vi "CONF digital do task.vi"(6 "Route array":i32[](array[numeric])=[1, 2, 3, 4, 5, 6, 7, 8], 8 "error in (no error)":errorcluster, 9 "Reorder config (F)":bool=TRUE, 10 "AI HW conf array in":T1[](array[typedef]), 11 "Digital ref in":T2) -> (0 "error out":errorcluster, 2 "AI HW conf array out":T1[](array[typedef]), 3 "Digital ref out":T2)   [LabVIEW 2013]
uses:
  Kontrolki/KartaDAQ/CONF Digital Refnum.ctl
  Kontrolki/KartaDAQ/CONF AI HW config.ctl
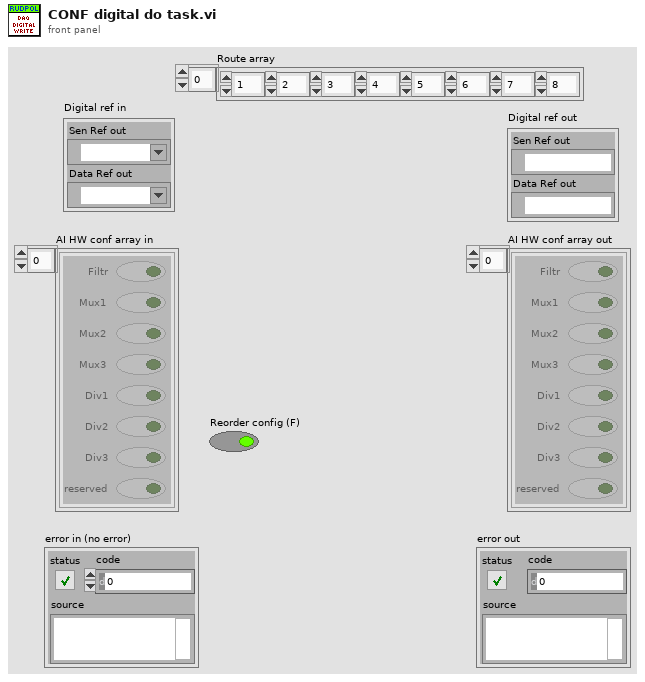
[diagram p1: front panel]
types:
  T1 = typedef "CONF AI HW config.ctl" = cluster{"Filtr":bool, "Mux1":bool, "Mux2":bool, "Mux3":bool, "Div1":bool, "Div2":bool, "Div3":bool, "reserved":bool}
  T2 = typedef "CONF Digital Refnum.ctl" = cluster{"Sen Ref out":refnum<k21>, "Data Ref out":refnum<k21>}
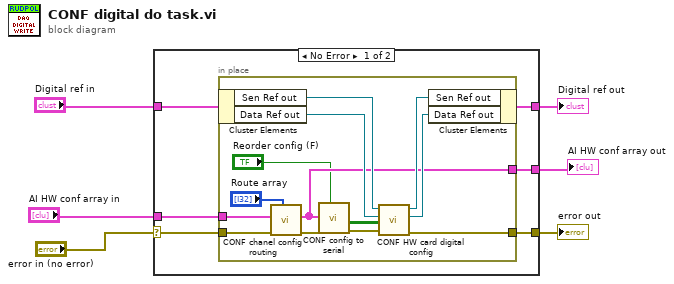
[diagram p0: block diagram]
diagram:
  n1 = case shown="No Error" "error in (no error)" {
    selector: "error in (no error)" -> [w9 w28]
    tunnel: "AI HW conf array in" -> [w8 w26]
    tunnel: [w10 w28] -> w6
    tunnel: "Digital ref in" -> [w12 w27]
    tunnel: [w11 w27] -> w4
    tunnel: [w7 w26] -> w1
    frame No Error {
      n2 = in-place {
        in-place-border: [w21] -> w10
        in-place-border: w9 -> [w20]
        in-place-border: w8 -> [w19]
        in-place-border: [w15] -> w7
        n3 = in-place-cluster #1(w12) -> ("Sen Ref out"=w25:refnum<k21>, "Data Ref out"=w24:refnum<k21>)
        n4 = call "CONF chanel config routing.vi"("Route array"="Route array", "error in (no error)"=w20, "AI HW conf array in"=w19) -> ("error out"=w17:errorcluster, "AI HW conf array out"=w15:T1[])  [unwired: 7 in]
        n5 = call "CONF config to serial.vi"("Reorder config"="Reorder config (F)", "error in (no error)"=w17, "AI HW conf array"=w15) -> ("error out"=w16:errorcluster, "Config serial out"=w14:bool[][])  [unwired: 6 in, 1 out]
        n6 = call "CONF HW card digital config.vi"("error in (no error)"=w16, "Config serial in"=w14, "DATA task in"=w24, "Enable task in"=w25) -> ("error out"=w21:errorcluster, "DATA task out"=w22:refnum<k21>, "Enable task out"=w23:refnum<k21>)  [unwired: 3 in, 2 out]
        n7 = in-place-cluster #1("Sen Ref out"=w23, "Data Ref out"=w22) -> (w11:T2)
      }
    }
    frame Error {
    }
  }
  "error out" <- w6
  "Digital ref out" <- w4
  "AI HW conf array out" <- w1
